vi "clear queues.vi"(8 "error in (no error)":errorcluster, 11 "queues":T1) -> (0 "error out":errorcluster, 3 "output device queues":T1)   [LabVIEW 2016]
uses:
  data.ctl
  device/device.ctl
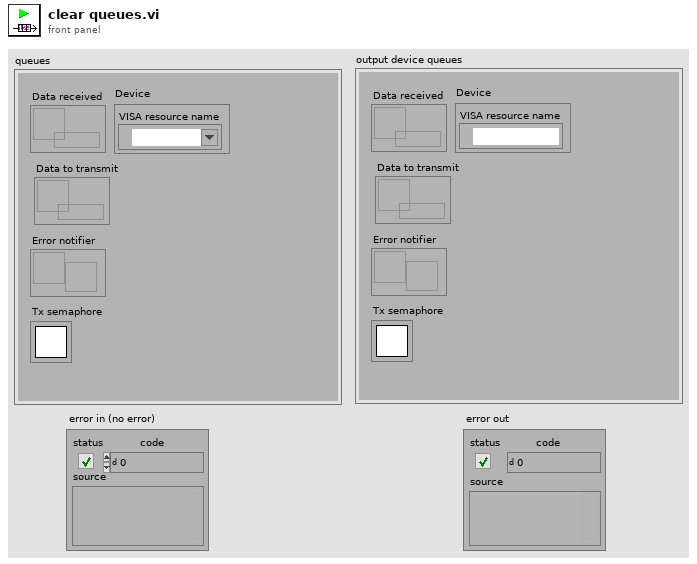
[diagram p1: front panel]
types:
  T1 = typedef "data.ctl" = cluster{"Data received":refnum<queue>, "Data to transmit":refnum<queue>, "Error notifier":refnum<notifier>, "Tx semaphore":T2, "Device":T3}
  T2 = typedef "Semaphore RefNum" = refnum<k1>
  T3 = typedef "device.ctl" = cluster{"VISA resource name":refnum<visa-resource-name>}
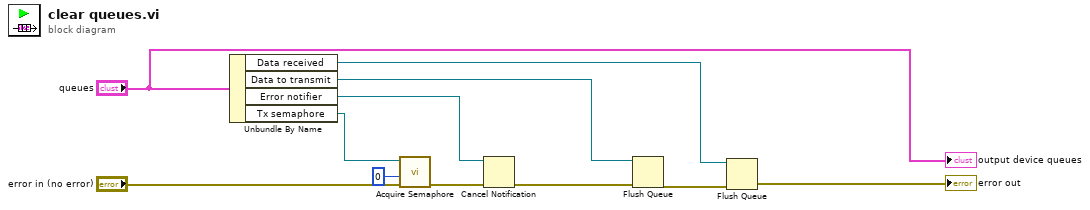
[diagram p0: block diagram]
diagram:
  n1 = Unbundle By Name("queues") -> ("Data received"=w4:refnum<queue>, "Data to transmit"=w6:refnum<queue>, "Error notifier"=w7:refnum<notifier>, "Tx semaphore"=w11:T2)
  n2 = call <vilib>:"Acquire Semaphore.vi"("error in (no error)"="error in (no error)", "ms timeout (-1)"=0, "semaphore"=w11) -> ("error out"=w8:errorcluster)  [unwired: 2 in, 2 out]
  n3 = Cancel Notification(0:w7, 3:w8) -> (11:w5:errorcluster)  [unwired: 2 out]
  n4 = Flush Queue(queue=w6, error in (no error)=w5) -> (error out=w3:errorcluster)  [unwired: 2 out]
  n5 = Flush Queue(queue=w4, error in (no error)=w3) -> (error out=→"error out":errorcluster)  [unwired: 2 out]
  "output device queues" <- "queues"
